vi "GetListInstruments.vi"(11 "Instrument type":T1(ring)) -> (3 "Instruments":string[](array[string]))   [LabVIEW 2018]
uses:
  InstrumentSetup.vi
  InstrControl.lvclass
panel:
  out "Instrument type 3":T1(ring)
  out "Instrument type 2":T1(ring)
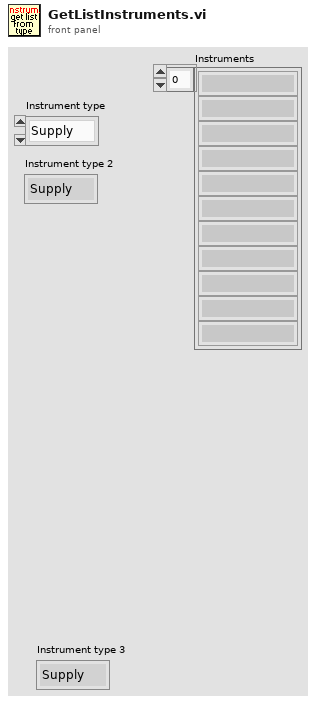
[diagram p1: front panel]
types:
  T1 = enum16{"Supply", "LCR", "Switching", "Multimeter"}
  T2 = cluster{"KE 2410":cluster{"Instrument name":string, "GPIB address":string, "Instrument type":u16}, "KE 6517":cluster{"Instrument name":string, "GPIB address":string, "Instrument type":u16}, "KE 487":cluster{"Instrument name":string, "GPIB address":string, "Instrument type":u16}, "KE 487_2":cluster{"Instrument name":string, "GPIB address":string, "Instrument type":u16}, "KE 236":cluster{"Instrument name":string, "GPIB address":string, "Instrument type":u16}, "WK 6440B":cluster{"Instrument name":string, "GPIB address":string, "Instrument type":u16}, "WK 6425":cluster{"Instrument name":string, "GPIB address":string, "Instrument type":u16}, "Pickering Matrix":cluster{"Instrument name":string, "GPIB address":string, "Instrument type":u16}, "KE 2000":cluster{"Instrument name":string, "GPIB address":string, "Instrument type":u16}, "KE 2657A":cluster{"Instrument name":string, "GPIB address":string, "Instrument type":u16}, "Prague Pickering Matrix":cluster{"Instrument name":string, "GPIB address":string, "Instrument type":u16}, "HP 4284A":cluster{"Instrument name":string, "GPIB address":string, "Instrument type":u16}}
  T3 = cluster{"Instrument name":string, "GPIB address":string, "Instrument type":u16}[]
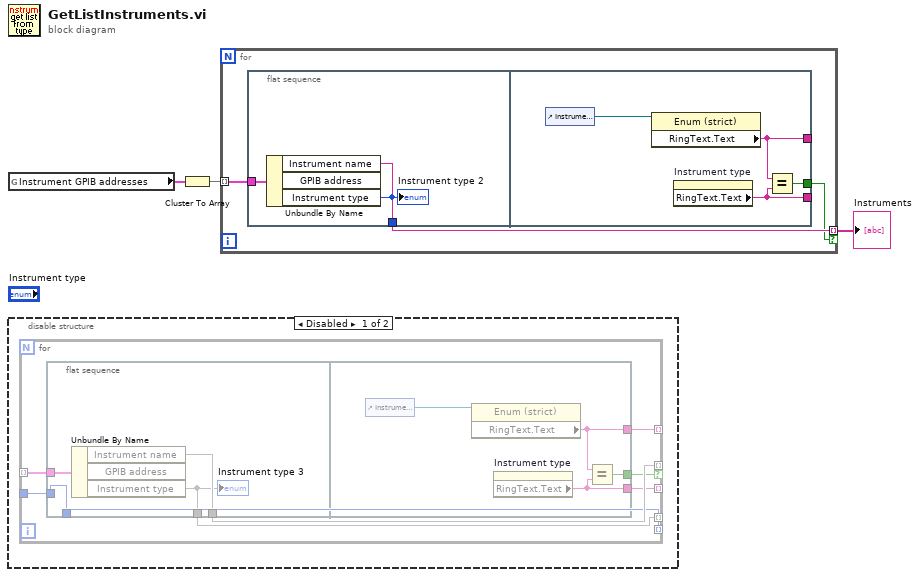
[diagram p0: block diagram]
diagram:
  n1 = global read "InstrumentSetup.vi" "Instrument GPIB addresses"() -> (w3:T2)
  n2 = disable-structure shown="Disabled" {
    frame Disabled {
      n3 = for {
        tunnel: _ -> [w11] mode=indexing
        tunnel: _ -> [w10]
        tunnel: [w9] -> _ mode=indexing if=w8
        tunnel: [w7] -> _ mode=indexing
        tunnel: [w6] -> _ mode=indexing
        tunnel: [w5] -> _ mode=indexing
        tunnel: [w4] -> _ mode=indexing
        n4 = flat-sequence {
          tunnel: w11 -> [w15]
          tunnel: w10 -> [w12]
          tunnel: [w14] -> w9
          tunnel: [w13] -> w7
          tunnel: [w12] -> w6
          tunnel: [w18] -> w8
          tunnel: [w17] -> w5
          tunnel: [w16] -> w4
          frame #0 {
            n5 = Unbundle By Name(w15) -> ("Instrument name"=w14, "Instrument type"=w13)  [unwired: 1 out]
            "Instrument type 3" <- w13
          }
          frame #1 {
            n6 = control-ref of="Instrument type 3"() -> (w19:refnum<vi>)
            n7 = property class="Enum (strict)"(reference=w19) -> ("RingText.Text"=w17:string)  [unwired: 1 in, 2 out]
            n8 = property on="Instrument type" class="Enum (strict)"() -> ("RingText.Text"=w16:string)  [unwired: 2 in, 2 out]
            n9 = Equal?(x=w17, y=w16) -> (x = y?=w18:bool)
          }
        }
      }
    }
    frame Enabled {
    }
  }
  n10 = Cluster To Array(cluster=w3) -> (array=w2:T3)
  n11 = for {
    tunnel: w2 -> [w22] mode=indexing
    tunnel: [w21] -> w1 mode=indexing if=w20
    n12 = flat-sequence {
      tunnel: w22 -> [w25]
      tunnel: [w24] -> w21
      tunnel: [w23] -> _
      tunnel: [w28] -> w20
      tunnel: [w27] -> _
      tunnel: [w26] -> _
      frame #0 {
        n13 = Unbundle By Name(w25) -> ("Instrument name"=w24:string, "Instrument type"=w23:u16)  [unwired: 1 out]
        "Instrument type 2" <- w23
      }
      frame #1 {
        n14 = control-ref of="Instrument type 2"() -> (w29:refnum<vi>)
        n15 = property class="Enum (strict)"(reference=w29) -> ("RingText.Text"=w27:string)  [unwired: 1 in, 2 out]
        n16 = property on="Instrument type" class="Enum (strict)"() -> ("RingText.Text"=w26:string)  [unwired: 2 in, 2 out]
        n17 = Equal?(x=w27, y=w26) -> (x = y?=w28:bool)
      }
    }
  }
  "Instruments" <- w1
